vi "CleanUp Diagram.vi"(8 "error in (no error)":errorcluster, 10 "Top Level Diagram":refnum<vi>, 11 "Module Loop in":refnum<class "Module Loop.lvclass">) -> (0 "error out":errorcluster, 3 "Module Loop out":refnum<class "Module Loop.lvclass">)   [LabVIEW 2015, in "Module Loop.lvclass"]
uses:
  Module Loop.lvclass
  Structures/Structures.lvclass/Structures.ctl
  Module Loop.lvclass/Module Loop.ctl
  Structures/Read Structure.vi
  Read Loop Structure.vi
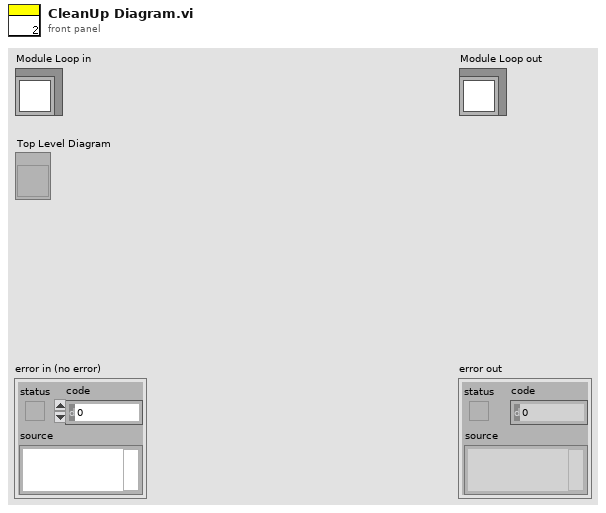
[diagram p1: front panel]
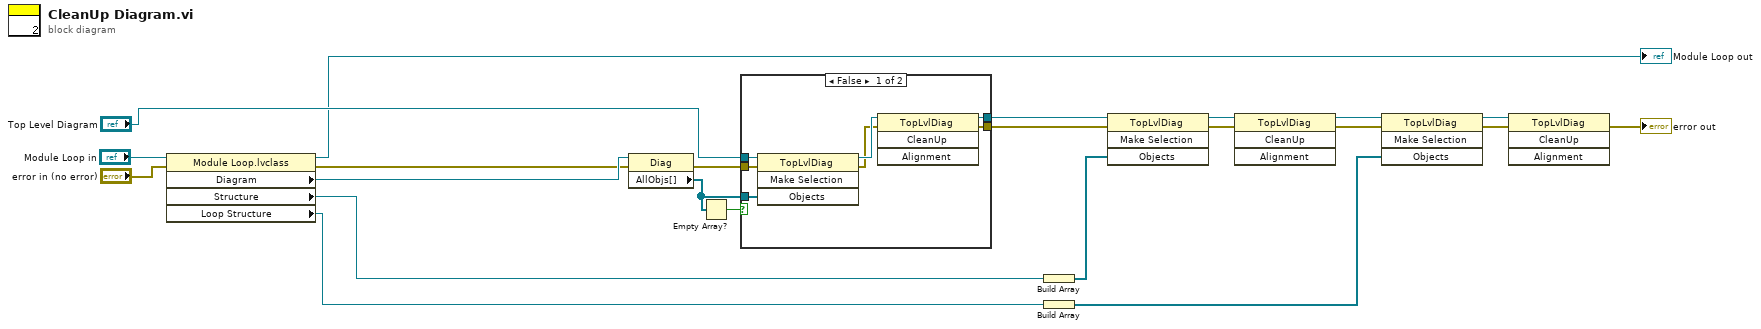
[diagram p0: block diagram]
diagram:
  n1 = property class="Module Loop.lvclass"(reference="Module Loop in", error in="error in (no error)") -> (reference out=→"Module Loop out":refnum<class "Module Loop.lvclass">, error out=w1:errorcluster, "Diagram"=w22:refnum<vi>, "Structure"=w2:refnum<vi>, "Loop Structure"=w4:refnum<vi>)
  n2 = property class="Diag"(reference=w22, error in=w1) -> (error out=w21:errorcluster, "AllObjs[]"=w17:refnum<vi>[])  [unwired: 1 out]
  n3 = Empty Array?(array=w17) -> (empty?=w16:bool)
  n4 = case shown="False" w16 {
    tunnel: "Top Level Diagram" -> [w29 w30]
    tunnel: w21 -> [w26 w31]
    tunnel: [w25 w31] -> w3
    tunnel: [w24 w30] -> w19
    tunnel: w17 -> [w23 _]
    frame False {
      n5 = invoke class="TopLvlDiag" method="Make Selection"(reference=w29, error in=w26, "Objects"=w23) -> (reference out=w28:refnum<vi>, error out=w27:errorcluster)  [unwired: 1 in, 2 out]
      n6 = invoke class="TopLvlDiag" method="CleanUp"(reference=w28, error in=w27) -> (reference out=w24:refnum<vi>, error out=w25:errorcluster)  [unwired: 2 in, 2 out]
    }
    frame True {
    }
  }
  n7 = Build Array(w2) -> (w15:refnum<vi>[])
  n8 = Build Array(w4) -> (w10:refnum<vi>[])
  n9 = invoke class="TopLvlDiag" method="Make Selection"(reference=w19, error in=w3, "Objects"=w15) -> (reference out=w18:refnum<vi>, error out=w20:errorcluster)  [unwired: 1 in, 2 out]
  n10 = invoke class="TopLvlDiag" method="CleanUp"(reference=w18, error in=w20) -> (reference out=w11:refnum<vi>, error out=w12:errorcluster)  [unwired: 2 in, 2 out]
  n11 = invoke class="TopLvlDiag" method="Make Selection"(reference=w11, error in=w12, "Objects"=w10) -> (reference out=w14:refnum<vi>, error out=w13:errorcluster)  [unwired: 1 in, 2 out]
  n12 = invoke class="TopLvlDiag" method="CleanUp"(reference=w14, error in=w13) -> (error out=→"error out":errorcluster)  [unwired: 2 in, 3 out]
